vi "PID Calculate I.vi"(0 "Error":dbl, 5 "Last Error":dbl, 7 "From Shift Register":dbl, 9 "Gains":cluster{"P":dbl, "I":dbl, "D":dbl}, 11 "Change in Time":u32) -> (4 "Output":dbl, 8 "To Shift Register":dbl)   [LabVIEW 2014]
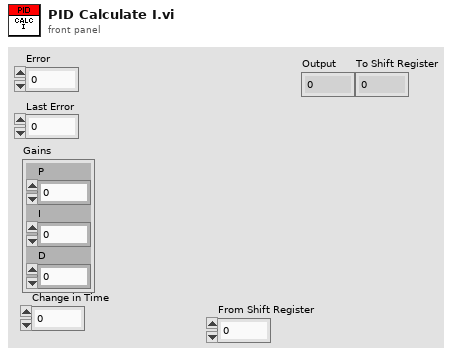
[diagram p1: front panel]
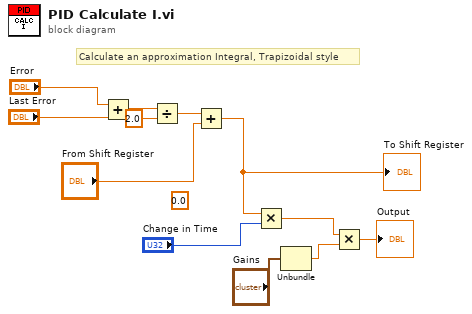
[diagram p0: block diagram]
diagram:
  (unwired) 0.0
  # "Calculate an approximation Integral, Trapizoidal style"
  n1 = Add(x="Error", y="Last Error") -> (x+y=w9:dbl)
  n2 = Divide(x=w9, y=2.0) -> (x/y=w3:dbl)
  n3 = Add(x=w3, y="From Shift Register") -> (x+y=w2:dbl)
  "To Shift Register" <- w2
  n4 = Multiply(x=w2, y="Change in Time") -> (x*y=w5:dbl)
  n5 = Unbundle("Gains") -> ("I"=w6:dbl)  [unwired: 2 out]
  n6 = Multiply(x=w5, y=w6) -> (x*y=→"Output":dbl)
